vi "dsc9513SetCMR.vi"(8 "error in":errorcluster, 10 "cmr":T1, 11 "board":i16) -> (0 "error out":errorcluster, 3 "boardOut":i16)   [LabVIEW 2011, in "Diamond Universal Driver.lvlib"]
doc: "Configures the Counter Mode Register for a counter on GPIO-MM-11 or GPIO-MM-12. The Counter Mode Register for a counter must be configured before that counter can be used."
uses:
  Diamond Universal Driver.lvlib
  Controls/dscqmmcmr.ctl
  Controls/QMM Gating Control.ctl
  Controls/counter source.ctl
  Controls/Output Control.ctl
  Controls/error codes.ctl
  Instruments/WL OPC/Support/dlls/dscud.dll
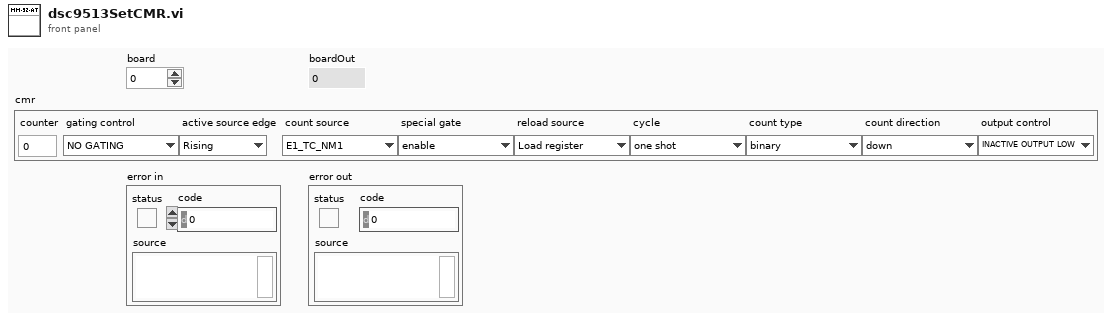
[diagram p1: front panel]
types:
  T1 = typedef "dscqmmcmr.ctl" = cluster{"counter":u8, "gating control":T2, "active source edge":enum8{"Rising", "Falling"}, "count source":T3, "special gate":enum8{"enable", "disable"}, "reload source":enum8{"Load register", "Load or hold register"}, "cycle":enum8{"one shot", "recycle"}, "count type":enum8{"binary", "BCD"}, "count direction":enum8{"down", "up"}, "output control":T4}
  T2 = typedef "Diamond Universal Driver.lvlib/QMM Gating Control.ctl" = enum8{"NO GATING", "ACTIVE HIGH TC NM1", "ACTIVE HIGH LEVEL GATE NP1", "ACTIVE HIGH LEVEL GATE NM1", "ACTIVE HIGH LEVEL GATE N", "ACTIVE LOW LEVEL GATE N", "ACTIVE HIGH EDGE GATE N", "ACTIVE LOW EDGE GATE N"}
  T3 = typedef "Diamond Universal Driver.lvlib/counter source.ctl" = enum8{"E1_TC_NM1", "SRC1", "SRC2", "SRC3", "SRC4", "SRC5", "GATE1", "GATE2", "GATE3", "GATE4", "GATE5", "F1_4MHZ", "F2_400KHZ", "F3_40KHZ", "F4_4KHZ", "F5_400HZ"}
  T4 = typedef "Diamond Universal Driver.lvlib/Output Control.ctl" = enum8{"INACTIVE OUTPUT LOW", "ACTIVE HIGH PULSE ON TC", "TOGGLE ON TC", "INACTIVE OUTPUT HIGH", "ACTIVE LOW PULSE ON TC"}
  T5 = typedef "Diamond Universal Driver.lvlib/error codes.ctl" = enum8{"DE_NONE", "DE_HW_FAILURE", "DE_SW_FAILURE", "DE_HW_NOT_SUPPORTED", "DE_SW_NOT_SUPPORTED", "DE_INVALID_PARM", "DE_ALTERNATE_IN_PROGRESS", "DE_NONE_IN_PROGRESS", "DE_BUFFER_ROLLOVER", "DE_INVALID_ERROR_CODE", "DE_ALREADY_PAUSED", "DE_OVERFLOW", "DE_INVALID_FUNC", "DE_DSCUDH_INVALID", "DE_INVALID_BOARD", "DE_BOARD_LIMIT_REACHED", "DE_BOARD_BUSY", "DE_INVALID_WINDRVR_HANDLE", "DE_INVALID_WINDRVR_VERSION", "DE_BAD_WINDRVR_BOARD_INIT", "DE_OPERATION_TIMED_OUT", "DE_INVALID_WINDRVR_KP", "DE_THREAD_FAILURE"}
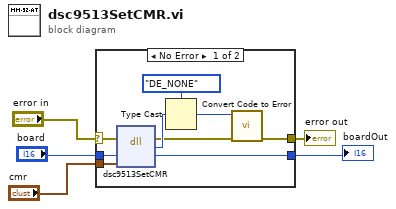
[diagram p0: block diagram]
diagram:
  n1 = case shown="No Error" "error in" {
    selector: "error in" -> [w11 w16]
    tunnel: "board" -> [w9 w15]
    tunnel: [w8 w15] -> w3
    tunnel: [w7 w16] -> w2
    tunnel: "cmr" -> [w6 _]
    frame No Error {
      n2 = dll-call lib="C:/Users/mrichardson/Documents/Web Based Version Control SW/Instruments/WL OPC/Support/dlls/dscud.dll" fn="dsc9513SetCMR"(error in=w11, "board"=w9, "dscqmm_cmr"=w6) -> (error out=w10:errorcluster, "error"=w12:u8, "board"=w8:i16)  [unwired: 3 in, 1 out]
      n3 = Type Cast(type=error_codes."DE_NONE" ("error codes"), x=w12) -> (*(type *) &x=w14:T5)
      n4 = call "Convert Code to Error.vi"("error in"=w10, "error codes"=w14) -> ("error out"=w7:errorcluster)  [unwired: 9 in]
    }
    frame Error {
    }
  }
  "boardOut" <- w3
  "error out" <- w2
